vi "Receive.vi"(11 "Base Event jettl in":refnum<class "Base Event jettl.lvclass">) -> (2 "Registration":refnum<event-registration>, 3 "Base Event jettl out":refnum<class "Base Event jettl.lvclass">)   [LabVIEW 2021, in "jettl.lvlib" / "Base Event jettl.lvlib" / "Base Event jettl.lvclass"]
uses:
  Base Event jettl.lvclass
  Msg Strategy/Msg Strategy.lvclass
  Base Event jettl.lvclass/Base Event jettl.ctl
  Self Event/Self Event.lvlib
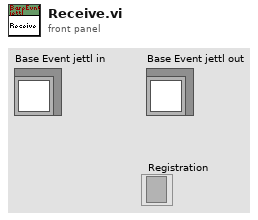
[diagram p1: front panel]
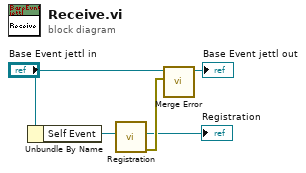
[diagram p0: block diagram]
diagram:
  n1 = Unbundle By Name("Base Event jettl in") -> ("Self Event"=w2:refnum<data-value>)
  n2 = call "Registration.vi"("Self Event"=w2) -> ("error out"=w3:errorcluster, "Registration"=→"Registration":refnum<event-registration>)  [unwired: 9 in]
  n3 = call-dynamic "Merge Error.vi"("Error"=w3, "Base Event jettl in"="Base Event jettl in") -> ("Base Event jettl out"=→"Base Event jettl out":refnum<class "Base Event jettl.lvclass">)  [unwired: 9 in]
